vi "Is_Path.vi"(0 "File_Path_In":path, 5 "File_Name":path=path "Library/text01.txt") -> (4 "File_Path_Out":path)   [LabVIEW 2021]
doc: "This VI Check if the user enter the path for the file or not. if not, it gives the default path."
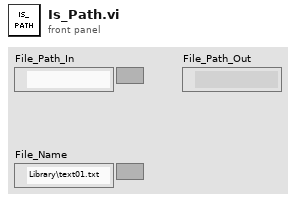
[diagram p1: front panel]
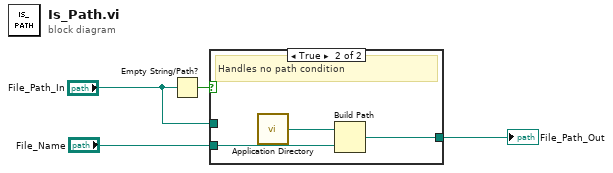
[diagram p0: block diagram]
diagram:
  n1 = Empty String/Path?(string/path="File_Path_In") -> (empty?=w3:bool)
  n2 = case shown="True" w3 {
    tunnel: [w5 w7] -> w1
    tunnel: "File_Path_In" -> [w5 _]
    tunnel: "File_Name" -> [_ w6]
    frame False {
      # "Handles User path condition"
    }
    frame True {
      # "Handles no path condition"
      n3 = call <vilib>:"Application Directory.vi"() -> ("Application Directory"=w8:path)
      n4 = Build Path(base path=w8, name or relative path=w6) -> (appended path=w7:path)
    }
  }
  "File_Path_Out" <- w1
